vi "ScpChGetRanges.vi"(8 "error in (no error)":errorcluster, 10 "wCh in":u16, 11 "hDevice in":u32) -> (0 "error out":errorcluster, 1 "pList out":dbl[](array[numeric]), 2 "dwRangeCount":u32, 3 "hDevice out":u32)   [LabVIEW 2018, in "LibTiePie.lvlib"]
uses:
  LibTiePie.lvlib
  LabViewHS4/libtiepie.dll
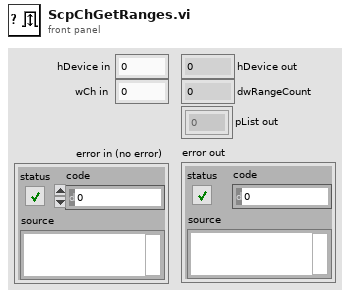
[diagram p1: front panel]
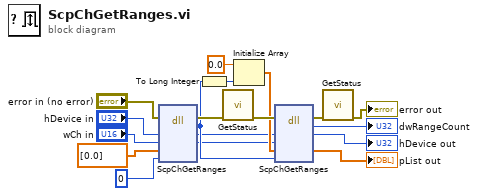
[diagram p0: block diagram]
diagram:
  n1 = dll-call lib="C:/Users/cwaha/Documents/LabViewHS4/libtiepie.dll" fn="ScpChGetRanges"(error in="error in (no error)", "hDevice"="hDevice in", "wCh"="wCh in", "pList"=dbl[] [0.0] ("NULL"), "dwRangeCount"=u32 0 ("NULL")) -> (error out=w16:errorcluster, "dwRangeCount"=w10:u32, "hDevice"=w9:u32, "wCh"=w8:u16)  [unwired: 4 in, 1 out]
  n2 = To Long Integer(number=w10) -> (32bit integer=w18:i32)
  n3 = call "GetStatus.vi"("error in (no error)"=w16) -> ("error out"=w12:errorcluster)  [unwired: 10 in]
  n4 = Initialize Array(0.0 ("element"), w18) -> (w11:dbl[])
  n5 = dll-call lib="C:/Users/cwaha/Documents/LabViewHS4/libtiepie.dll" fn="ScpChGetRanges"(error in=w12, "hDevice"=w9, "wCh"=w8, "pList"=w11, "dwRangeCount"=w10) -> (error out=w13:errorcluster, "dwRangeCount"=→"dwRangeCount":u32, "hDevice"=→"hDevice out":u32, "pList"=→"pList out":dbl[])  [unwired: 4 in, 1 out]
  n6 = call "GetStatus.vi"("error in (no error)"=w13) -> ("error out"=→"error out":errorcluster)  [unwired: 10 in]
